vi "TempLimitsConfigurables_SubVI.vi"(10 "TempMin":i32, 11 "TempMax":i32) -> (3 "RandomTemp":dbl)   [LabVIEW 2019]
doc: "Genera una temperatura entre els límits definits"
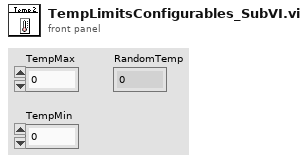
[diagram p1: front panel]
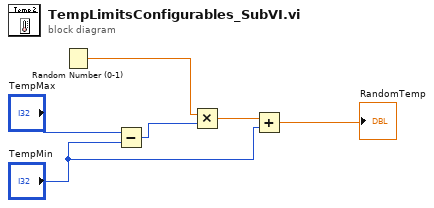
[diagram p0: block diagram]
diagram:
  n1 = Random Number (0-1)() -> (number: 0 to 1=w4:dbl)
  n2 = Subtract(x="TempMax", y="TempMin") -> (x-y=w5:i32)
  n3 = Multiply(x=w4, y=w5) -> (x*y=w2:dbl)
  n4 = Add(x=w2, y="TempMin") -> (x+y=→"RandomTemp":dbl)
